vi "Remove File Extensions.vi"(10 "Extensions (all library extensions)":string[](array[string])=[".lvclass", ".lvlib", ".xctl", ".xnode", ".lvsc", ".lvlibp"], 11 "File name in":string) -> (3 "File name without extension":string)   [LabVIEW 2013, in "UserTBModuleDecideFeatures.lvclass"]
uses:
  UserTBModuleDecideFeatures.lvclass
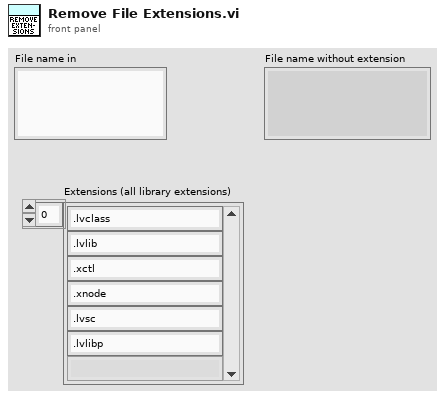
[diagram p1: front panel]
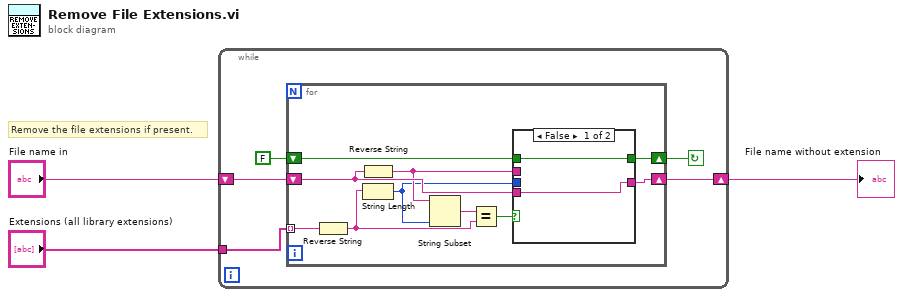
[diagram p0: block diagram]
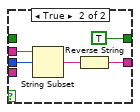
[diagram p2: hidden frame]
diagram:
  # "Remove the file extensions if present."
  n1 = while {
    tunnel: "Extensions (all library extensions)" -> [w6]
    shift-right: [w7] -> w2
    shift-left: "File name in" -> [w8]
    stop <- w5 continue-if-true
    n2 = for {
      tunnel: w6 -> [w11] mode=indexing
      shift-right: [w17] -> w7
      shift-left: w8 -> [w18]
      shift-right: [w10] -> w5
      shift-left: FALSE -> [w9]
      n3 = Reverse String(1:w11) -> (0:w12:string)
      n4 = Reverse String(1:w18) -> (0:w14:string)
      n5 = String Length(string=w12) -> (length=w13:i32)
      n6 = String Subset(string=w14, length (rest)=w13) -> (substring=w15:string)  [unwired: 1 in]
      n7 = Equal?(x=w15, y=w12) -> (x = y?=w16:bool)
      n8 = case shown="False" w16 {
        tunnel: [w20 w22] -> w17
        tunnel: w18 -> [w20 _]
        tunnel: w13 -> [_ w25]
        tunnel: w14 -> [_ w24]
        tunnel: [w19 TRUE] -> w10
        tunnel: w9 -> [w19 _]
        frame False {
        }
        frame True {
          n9 = String Subset(string=w24, offset (0)=w25) -> (substring=w23:string)  [unwired: 1 in]
          n10 = Reverse String(1:w23) -> (0:w22:string)
        }
      }
    }
  }
  "File name without extension" <- w2
